vi "InterruptHandler.vi"(8 "error in (no error)":errorcluster, 11 "mbedSerial in":refnum<class "SerialRPC.lvclass">) -> (0 "error out":errorcluster, 2 "Interrupt Name":string, 3 "mbedSerial out":refnum<class "SerialRPC.lvclass">)   [LabVIEW 2009]
uses:
  SerialRPC.lvclass
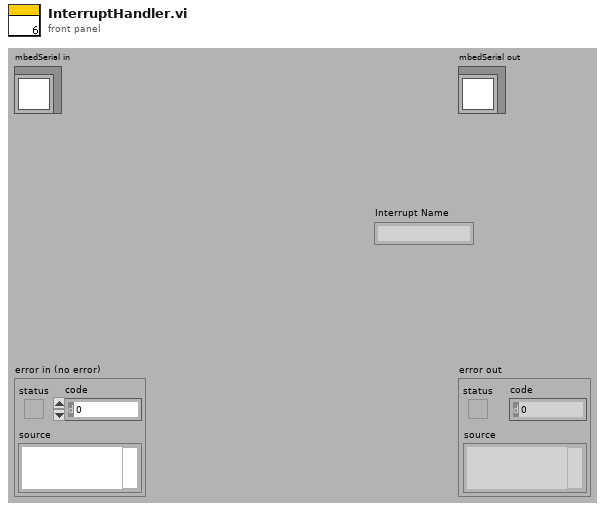
[diagram p1: front panel]
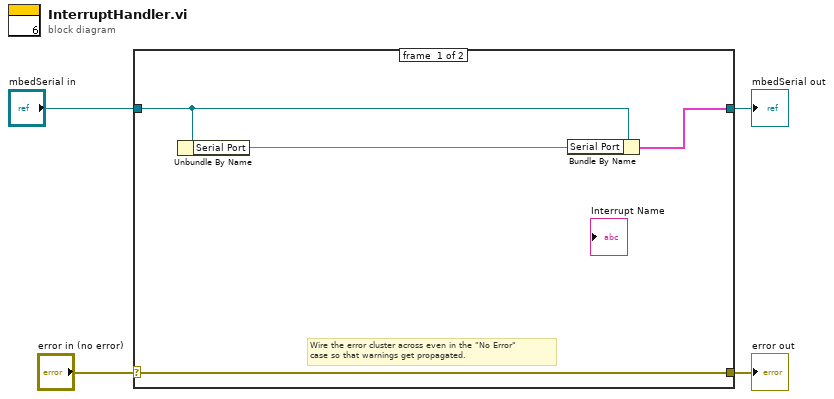
[diagram p0: block diagram]
diagram:
  n1 = case shown="No Error" "error in (no error)" {
    selector: "error in (no error)" -> [w8 w10]
    tunnel: [w8 w10] -> w3
    tunnel: [w6 w9] -> w1
    tunnel: "mbedSerial in" -> [w7 w9]
    frame #0 {
      # "Wire the error cluster across even in the \"No Error\"\ncase so that warnings get propagated."
      n2 = Unbundle By Name(w7) -> ("Serial Port"=w5)
      n3 = Bundle By Name(cluster=w7, "Serial Port"=w5) -> (w6:cluster{})
    }
    frame #1 {
    }
  }
  "error out" <- w3
  "mbedSerial out" <- w1
